vi "Celsius_to_Fahrenheit.vi"() -> ()   [LabVIEW 2019]
panel:
  out "Fahrenheit":dbl
  in  "Celsius":dbl
  # "Convert the temperature from Celsius to Fahrenheit"
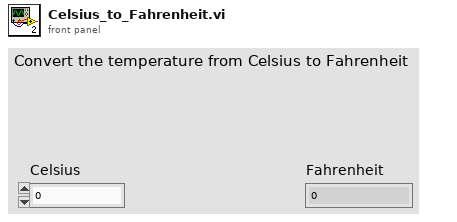
[diagram p1: front panel]
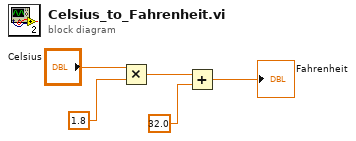
[diagram p0: block diagram]
diagram:
  n1 = Multiply(x="Celsius", y=1.8) -> (x*y=w3:dbl)
  n2 = Add(x=w3, y=32.0) -> (x+y=→"Fahrenheit":dbl)
